vi "FTW-ScheduledJob-SyncToSystemClock-Construct.vi"(0 "Scheduled Job Identity":string, 5 "Scheduled Period":i32=100 format="%d msec", 7 "Offset from Clock Multiple":i32 format="%d msec", 9 "Iterations (-1 to loop forever)":i32=-1 format="%d iterations", 11 "error in":errorcluster) -> (4 "Scheduled Job Synchronized to System Clock":refnum<class "FTW-ScheduledJob-SyncToSystemClock.lvclass">, 15 "error out":errorcluster)   [LabVIEW 2015, in "FTW-ScheduledJob-SyncToSystemClock.lvclass"]
uses:
  FTW-ScheduledJob-SyncToSystemClock.lvclass
  FTW-ScheduledJob.lvclass
panel:
  in  "Job":string
  # "Inputs"
  # "Outputs"
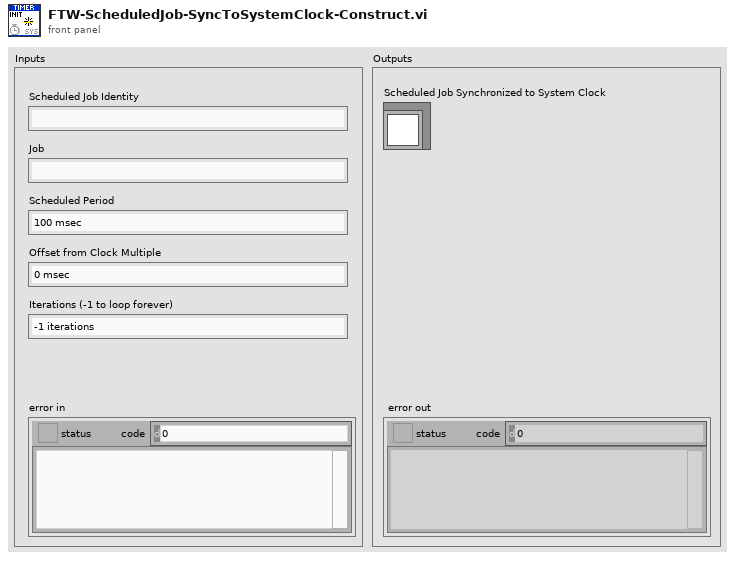
[diagram p1: front panel]
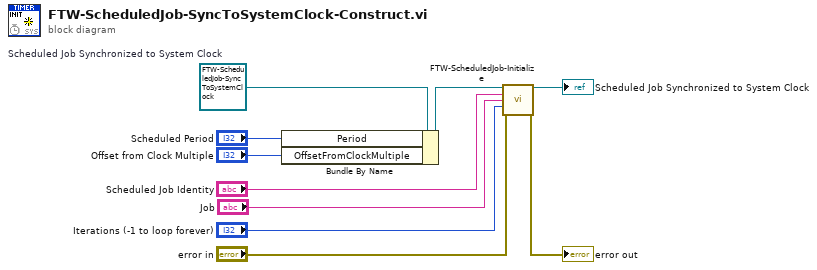
[diagram p0: block diagram]
diagram:
  w4 = refnum<class "FTW-ScheduledJob-SyncToSystemClock.lvclass"> refnum  # Scheduled Job Synchronized to System Clock
  n1 = Bundle By Name(cluster=w4, "Period"="Scheduled Period", "OffsetFromClockMultiple"="Offset from Clock Multiple") -> (w3:refnum<class "FTW-ScheduledJob-SyncToSystemClock.lvclass">)
  n2 = call "FTW-ScheduledJob-Initialize.vi"("FTW Scheduled Job"=w3, "Identity"="Scheduled Job Identity", "Job"="Job", "Iterations (-1 to loop forever)"="Iterations (-1 to loop forever)", "error in"="error in") -> ("FTW Scheduled Job out"=→"Scheduled Job Synchronized to System Clock":refnum<class "FTW-ScheduledJob-SyncToSystemClock.lvclass">, "error out"=→"error out":errorcluster)  [unwired: 9 in]
